vi "Create lvlib Folder.vi"(9 "Template Library File Path":path, 10 "Active Project":refnum<vi>) -> (0 "error out":errorcluster, 2 "Created Library File Path":path)   [LabVIEW 2025, in "_Template.lvlib" / "_Template.lvclass"]
uses:
  _Template.lvclass
  _Template.lvclass/_Template.ctl
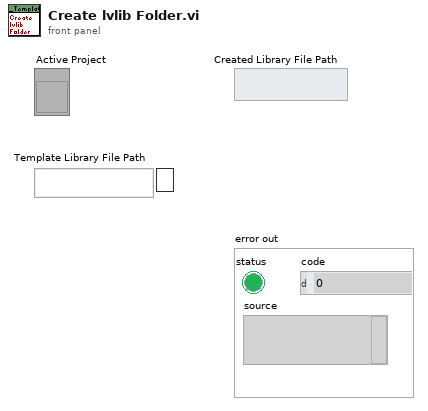
[diagram p1: front panel]
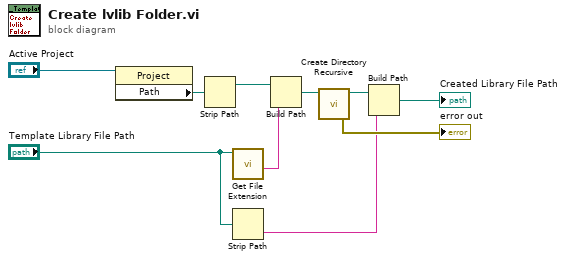
[diagram p0: block diagram]
diagram:
  n1 = property class="Project"(reference="Active Project") -> ("Path"=w7:path)  [unwired: 1 in, 2 out]
  n2 = Strip Path(path=w7) -> (stripped path=w10:path)  [unwired: 1 out]
  n3 = call <vilib>:"Get File Extension.vi"("file"="Template Library File Path") -> ("filename without extension"=w6:string)  [unwired: 6 in, 4 out]
  n4 = Strip Path(path="Template Library File Path") -> (name=w1:string)  [unwired: 1 out]
  n5 = Build Path(base path=w10, name or relative path=w6) -> (appended path=w4:path)
  n6 = call <vilib>:"Create Directory Recursive.vi"("directory"=w4) -> ("error out"=→"error out":errorcluster, "directory copy"=w3:path)  [unwired: 4 in, 1 out]
  n7 = Build Path(base path=w3, name or relative path=w1) -> (appended path=→"Created Library File Path":path)
